vi "BUILD_post build add to repo timing.vi"() -> ()   [LabVIEW 2013]
panel:
  out "error out":errorcluster
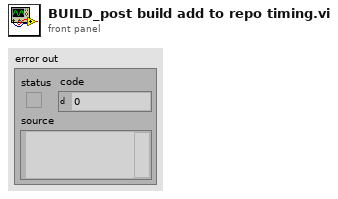
[diagram p1: front panel]
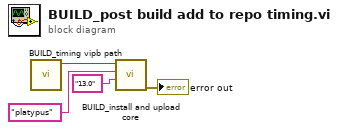
[diagram p0: block diagram]
diagram:
  n1 = call "BUILD_timing vipb path.vi"() -> ("appended path"=w1:path)  [unwired: 11 in]
  n2 = call "BUILD_install and upload core.vi"("LabVIEW Version"="13.0", "Repository Name"="platypus", "appended path"=w1) -> ("error out"=→"error out":errorcluster)  [unwired: 8 in]
